vi "sub ch-val-global.vi"(7 "Relay":T1=enum."R_in6", 8 "error in (no error)":errorcluster, 11 "onoff":bool) -> (0 "error out":errorcluster)   [LabVIEW 2019]
uses:
  cDAQ-9476 DO/cnt_Relay.ctl
  cDAQ-9476 DO/cnt_do.ctl
  Durability/common/cmd_timecheck.ctl
  Durability/common/Global 1.vi
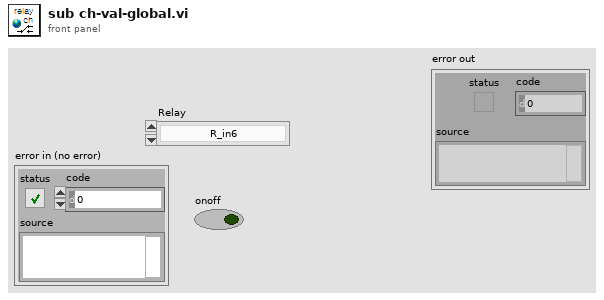
[diagram p1: front panel]
types:
  T1 = typedef "cnt_Relay.ctl" = enum32{"R_Load", "R_out1", "R_out2", "R_out3", "R_out4", "R_out5", "R_out6", "R8", "R9", "R10", "R11", "R12", "R13", "R14", "R15", "R16", "R_in1", "R_in2", "R_in3", "R_in4", "R_in5", "R_in6", "R23", "R24", "R25", "R26", "R27", "R_red", "R_yellow", "R_green", "R_buz", "R_purple"}
  T2 = typedef "cmd_timecheck.ctl" = enum16{"Group start", "Group end", "Grout dt", "Ch start", "Ch end", "Ch dt", "init", "NF start", "NF stop", "idrc start", "idrc stop", "scope start", "scope stop", "ao start", "ao stop", "relay start", "relay stop", "NF read start", "NF read stop", "NF set start", "NF set stop", "idrc level start", "idrc level stop", "scope trig start", "scope trig stop", "relay dischar star", "relay dischar stop", "data process start", "data process stop", "ch-relay on start", "ch-relay on stop", "hw set start", "hw set stop", "pwr-in on start", "pwr-in on stop", "pwr-out on start", "pwr-out on stop", "ao on start", "ao on stop", "ao 0v start", "ao 0v stop", "pwr-in off start", "pwr-in off stop", "relay-all off start", "relay-all off stop", "pwr-out off start", "pwr-out off stop", "discharge start", "discharge stop", "950 read start", "950 read stop"}
  T3 = typedef "cnt_do.ctl" = enum16{"open", "initial", "update", "run", "close"}
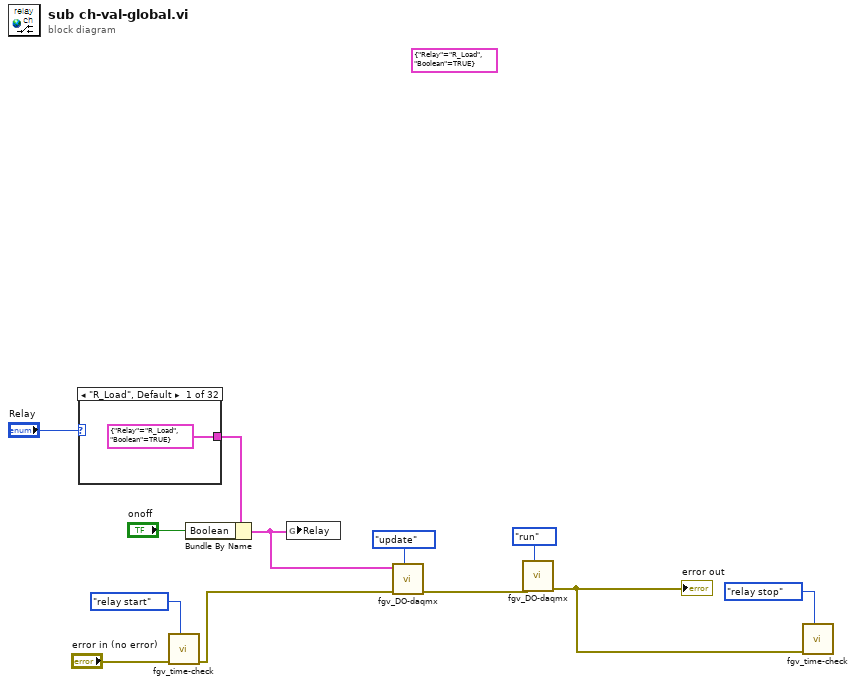
[diagram p0: block diagram]
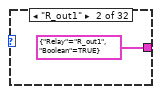
[diagram p2: hidden frame]
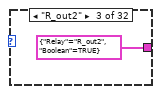
[diagram p3: hidden frame]
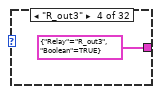
[diagram p4: hidden frame]
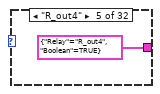
[diagram p5: hidden frame]
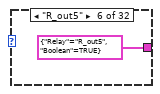
[diagram p6: hidden frame]
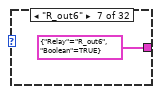
[diagram p7: hidden frame]
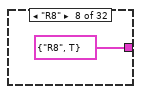
[diagram p8: hidden frame]
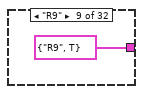
[diagram p9: hidden frame]
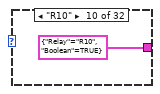
[diagram p10: hidden frame]
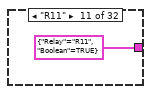
[diagram p11: hidden frame]
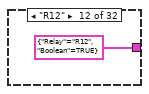
[diagram p12: hidden frame]
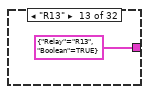
[diagram p13: hidden frame]
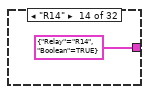
[diagram p14: hidden frame]
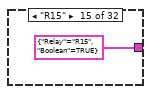
[diagram p15: hidden frame]
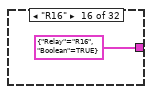
[diagram p16: hidden frame]
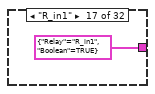
[diagram p17: hidden frame]
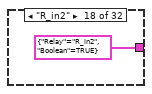
[diagram p18: hidden frame]
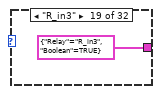
[diagram p19: hidden frame]
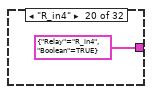
[diagram p20: hidden frame]
diagram:
  (unwired) cluster{"Relay":T1, "Boolean":bool} {"Relay"=enum."R_Load", "Boolean"=TRUE} ("Relay")
  n1 = case shown="\"R_Load\", Default" "Relay" {
    tunnel: [cluster{"Relay":T1, "Boolean":bool} {"Relay"=enum."R_Load", "Boolean"=TRUE} ("Relay") cluster{"Relay":T1, "Boolean":bool} {"Relay"=enum."R_out1", "Boolean"=TRUE} ("Relay") cluster{"Relay":T1, "Boolean":bool} {"Relay"=enum."R_out2", "Boolean"=TRUE} ("Relay") cluster{"Relay":T1, "Boolean":bool} {"Relay"=enum."R_out3", "Boolean"=TRUE} ("Relay") cluster{"Relay":T1, "Boolean":bool} {"Relay"=enum."R_out4", "Boolean"=TRUE} ("Relay") cluster{"Relay":T1, "Boolean":bool} {"Relay"=enum."R_out5", "Boolean"=TRUE} ("Relay") cluster{"Relay":T1, "Boolean":bool} {"Relay"=enum."R_out6", "Boolean"=TRUE} ("Relay") cluster{"Relay":T1, "Boolean":bool} {"Relay"=enum."R8", "Boolean"=TRUE} ("Relay") cluster{"Relay":T1, "Boolean":bool} {"Relay"=enum."R9", "Boolean"=TRUE} ("Relay") cluster{"Relay":T1, "Boolean":bool} {"Relay"=enum."R10", "Boolean"=TRUE} ("Relay") cluster{"Relay":T1, "Boolean":bool} {"Relay"=enum."R11", "Boolean"=TRUE} ("Relay") cluster{"Relay":T1, "Boolean":bool} {"Relay"=enum."R12", "Boolean"=TRUE} ("Relay") cluster{"Relay":T1, "Boolean":bool} {"Relay"=enum."R13", "Boolean"=TRUE} ("Relay") cluster{"Relay":T1, "Boolean":bool} {"Relay"=enum."R14", "Boolean"=TRUE} ("Relay") cluster{"Relay":T1, "Boolean":bool} {"Relay"=enum."R15", "Boolean"=TRUE} ("Relay") cluster{"Relay":T1, "Boolean":bool} {"Relay"=enum."R16", "Boolean"=TRUE} ("Relay") cluster{"Relay":T1, "Boolean":bool} {"Relay"=enum."R_in1", "Boolean"=TRUE} ("Relay") cluster{"Relay":T1, "Boolean":bool} {"Relay"=enum."R_in2", "Boolean"=TRUE} ("Relay") cluster{"Relay":T1, "Boolean":bool} {"Relay"=enum."R_in3", "Boolean"=TRUE} ("Relay") cluster{"Relay":T1, "Boolean":bool} {"Relay"=enum."R_in4", "Boolean"=TRUE} ("Relay") cluster{"Relay":T1, "Boolean":bool} {"Relay"=enum."R_in5", "Boolean"=TRUE} ("Relay") cluster{"Relay":T1, "Boolean":bool} {"Relay"=enum."R_in6", "Boolean"=TRUE} ("Relay") cluster{"Relay":T1, "Boolean":bool} {"Relay"=enum."R23", "Boolean"=TRUE} ("Relay") cluster{"Relay":T1, "Boolean":bool} {"Relay"=enum."R24", "Boolean"=TRUE} ("Relay") cluster{"Relay":T1, "Boolean":bool} {"Relay"=enum."R25", "Boolean"=TRUE} ("Relay") cluster{"Relay":T1, "Boolean":bool} {"Relay"=enum."R26", "Boolean"=TRUE} ("Relay") cluster{"Relay":T1, "Boolean":bool} {"Relay"=enum."R27", "Boolean"=TRUE} ("Relay") cluster{"Relay":T1, "Boolean":bool} {"Relay"=enum."R_red", "Boolean"=TRUE} ("Relay") cluster{"Relay":T1, "Boolean":bool} {"Relay"=enum."R_yellow", "Boolean"=TRUE} ("Relay") cluster{"Relay":T1, "Boolean":bool} {"Relay"=enum."R_green", "Boolean"=TRUE} ("Relay") cluster{"Relay":T1, "Boolean":bool} {"Relay"=enum."R_buz", "Boolean"=TRUE} ("Relay") cluster{"Relay":T1, "Boolean":bool} {"Relay"=enum."R_purple", "Boolean"=TRUE} ("Relay")] -> w10
    frame "R_Load", Default {
    }
    frame "R_out1" {
    }
    frame "R_out2" {
    }
    frame "R_out3" {
    }
    frame "R_out4" {
    }
    frame "R_out5" {
    }
    frame "R_out6" {
    }
    frame "R8" {
    }
    frame "R9" {
    }
    frame "R10" {
    }
    frame "R11" {
    }
    frame "R12" {
    }
    frame "R13" {
    }
    frame "R14" {
    }
    frame "R15" {
    }
    frame "R16" {
    }
    frame "R_in1" {
    }
    frame "R_in2" {
    }
    frame "R_in3" {
    }
    frame "R_in4" {
    }
    frame "R_in5" {
    }
    frame "R_in6" {
    }
    frame "R23" {
    }
    frame "R24" {
    }
    frame "R25" {
    }
    frame "R26" {
    }
    frame "R27" {
    }
    frame "R_red" {
    }
    frame "R_yellow" {
    }
    frame "R_green" {
    }
    frame "R_buz" {
    }
    frame "R_purple" {
    }
  }
  n2 = call "fgv_time-check.vi"("cmd"=cmd_timecheck."relay start", "error in (no error)"="error in (no error)") -> ("error out"=w4:errorcluster)  [unwired: 8 in, 1 out]
  n3 = Bundle By Name(cluster=w10, "Boolean"="onoff") -> (w8:cluster{"Relay":T1, "Boolean":bool})
  n4 = global write "Global 1.vi" "Relay"(w8) -> ()
  n5 = call "fgv_DO-daqmx.vi"("cnt"=cnt_do."update", "error in"=w4, "Relay"=w8) -> ("error out"=w6:errorcluster)  [unwired: 8 in]
  n6 = call "fgv_DO-daqmx.vi"("cnt"=cnt_do."run", "error in"=w6) -> ("error out"=w2:errorcluster)  [unwired: 9 in]
  "error out" <- w2
  n7 = call "fgv_time-check.vi"("cmd"=cmd_timecheck."relay stop", "error in (no error)"=w2) -> ()  [unwired: 8 in, 2 out]
